vi "read.vi"(7 "timeout (ms)":i32, 8 "error in (no error)":errorcluster, 9 "number of channels":i32, 10 "block size":i32, 11 "FPGAWrapperMH120124FrameScan_PXI7813R in":refnum<class "FPGAWrapperMH120124FrameScan_PXI7813R.lvclass">) -> (0 "error out":errorcluster, 1 "channels raw data block":T1, 2 "FIFO full?":bool, 3 "FPGAWrapperMH120124FrameScan_PXI7813R out":refnum<class "FPGAWrapperMH120124FrameScan_PXI7813R.lvclass">, 4 "timed out?":bool)   [LabVIEW 2010, in "FPGAWrapperMH120124FrameScan_PXI7813R.lvclass"]
uses:
  FPGAWrapperMH120124FrameScan_PXI7813R.lvclass
  common/arrays/pixel_raw_data_array.ctl
  class_data.vi
  D:/Program Files/National Instruments/LabVIEW 2010/resource/objmgr/ni.dex.rc
panel:
  out "available elements remaining":i32
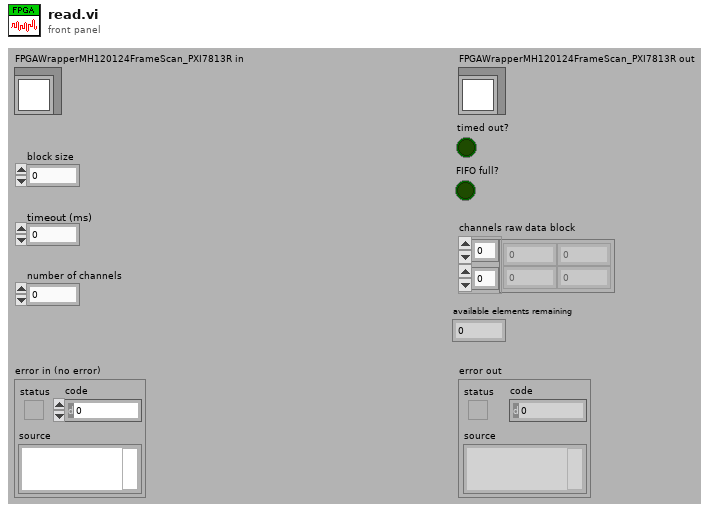
[diagram p1: front panel]
types:
  T1 = typedef "pixel_raw_data_array.ctl" = dbl[][]
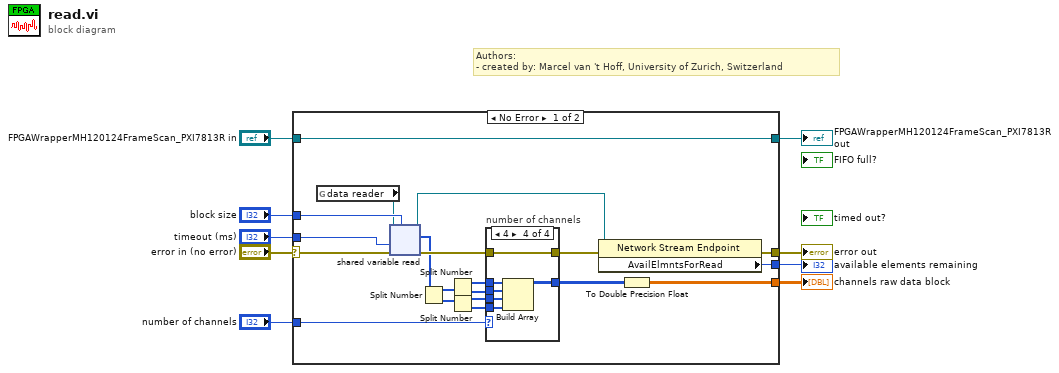
[diagram p0: block diagram]
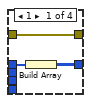
[diagram p2: hidden frame]
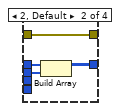
[diagram p3: hidden frame]
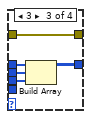
[diagram p4: hidden frame]
diagram:
  # "Authors: \n- created by: Marcel van 't Hoff, University of Zurich, Switzerland"
  n1 = case shown="No Error" "error in (no error)" {
    selector: "error in (no error)" -> [w28 w49]
    tunnel: [w22 w49] -> w8
    tunnel: [w29 w48] -> w7
    tunnel: "FPGAWrapperMH120124FrameScan_PXI7813R in" -> [w29 w48]
    tunnel: "block size" -> [w19 _]
    tunnel: "timeout (ms)" -> [w27 _]
    tunnel: "number of channels" -> [w25 _]
    tunnel: [w23 _] -> w2
    tunnel: [w20 _] -> w1
    frame No Error {
      n2 = global read "class_data.vi" "data reader"() -> (w11:refnum<k21>)
      n3 = shared-variable-read(w11, w28, w27, w19) -> (w10:refnum<k21>, w26:errorcluster, w18:u32[])  [unwired: 1 out]
      n4 = Split Number(x=w18) -> (hi(x)=w17:u16[], lo(x)=w12:u16[])
      n5 = Split Number(x=w17) -> (hi(x)=w16:u8[], lo(x)=w15:u8[])
      n6 = Split Number(x=w12) -> (hi(x)=w14:u8[], lo(x)=w13:u8[])
      n7 = case "number of channels" shown="4" w25 {
        tunnel: w16 -> [w32 w36 w38 w45]
        tunnel: [w31 w35 w41 w47] -> w24
        tunnel: [w30 w34 w40 w46] -> w21
        tunnel: w26 -> [w30 w34 w40 w46]
        tunnel: w15 -> [_ w33 w39 w44]
        tunnel: w14 -> [_ _ w37 w43]
        tunnel: w13 -> [_ _ _ w42]
        frame 1 {
          n8 = Build Array(w32) -> (w31:u8[][])
        }
        frame 2, Default {
          n9 = Build Array(w36, w33) -> (w35:u8[][])
        }
        frame 3 {
          n10 = Build Array(w38, w39, w37) -> (w41:u8[][])
        }
        frame 4 {
          n11 = Build Array(w45, w44, w43, w42) -> (w47:u8[][])
        }
      }
      n12 = property class="Network Stream Endpoint"(reference=w10, error in=w21) -> (error out=w22:errorcluster, "AvailElmntsForRead"=w20:i32)  [unwired: 1 out]
      n13 = To Double Precision Float(number=w24) -> (double precision float=w23:dbl[][])
    }
    frame Error {
    }
  }
  "error out" <- w8
  "FPGAWrapperMH120124FrameScan_PXI7813R out" <- w7
  "channels raw data block" <- w2
  "available elements remaining" <- w1
